vi "Split_Data.vi"(0 "Format_String (%s)":string="%s", 1 "Delimiter":string="\n", 5 "Data_In":string, 11 "Error_In":errorcluster) -> (4 "Split_Data_Out":string[](array[string]), 15 "Error_Out":errorcluster)   [LabVIEW 2021, in "File_Handler_Library.lvlib"]
doc: "This VI Splits string data and forms array"
uses:
  File_Handler_Library.lvlib
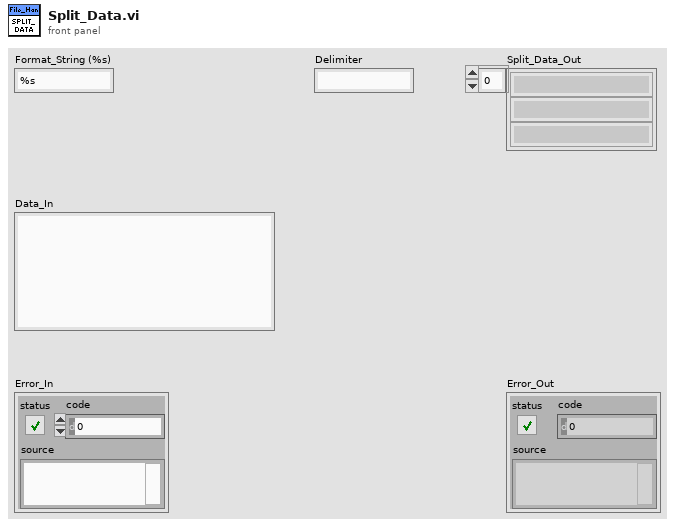
[diagram p1: front panel]
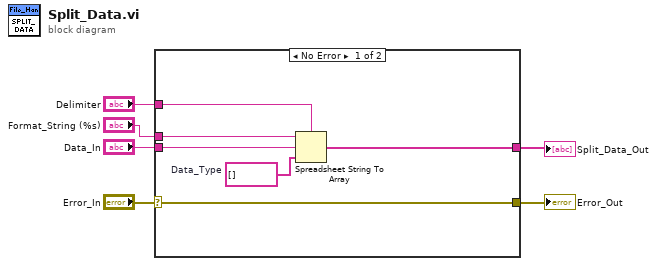
[diagram p0: block diagram]
diagram:
  n1 = case shown="No Error" "Error_In" {
    selector: "Error_In" -> [w11 w13]
    tunnel: [w11 w13] -> w5
    tunnel: "Format_String (%s)" -> [w10 _]
    tunnel: "Data_In" -> [w9 _]
    tunnel: "Delimiter" -> [w8 _]
    tunnel: [w7 _] -> w1
    frame No Error {
      w12 = string[] []  # Data_Type
      n2 = Spreadsheet String To Array(delimiter (Tab)=w8, format string=w10, spreadsheet string=w9, array type (2D Dbl)=w12) -> (array=w7:string[])
    }
    frame Error {
    }
  }
  "Error_Out" <- w5
  "Split_Data_Out" <- w1
